vi "DAQmx Create Channel (TEDS-AI-Position-RVDT).vi"(0 "task in":refnum<k21>, 1 "maximum value":dbl=70.0 format="%0.2f", 2 "minimum value":dbl=-70.0 format="%0.2f", 3 "voltage excitation wire mode":i32(ring)=4 items=["4-Wire"=4, "5-Wire"=5, "6-Wire"=6], 5 "physical channels":tag, 6 "voltage excitation source":i32(ring)=10200 items=["Internal"=10200, "External"=10167, "None"=10230], 7 "name to assign":string, 8 "voltage excitation value":dbl=1.0, 9 "units":i32(ring)=10146 items=["Degrees"=10146, "Radians"=10273, "From Custom Scale"=10065], 10 "voltage excitation frequency":dbl=2500.0, 11 "error in":errorcluster, 12 "custom scale name":tag) -> (4 "task out":refnum<k21>, 15 "error out":errorcluster)   [LabVIEW 2018]
doc: "Creates channel(s) that use an RVDT to measure angular position. You must configure the physical channel(s) with TEDS information to use this VI."
uses:
  nilvaiu.dll
panel:
  # "input limits"
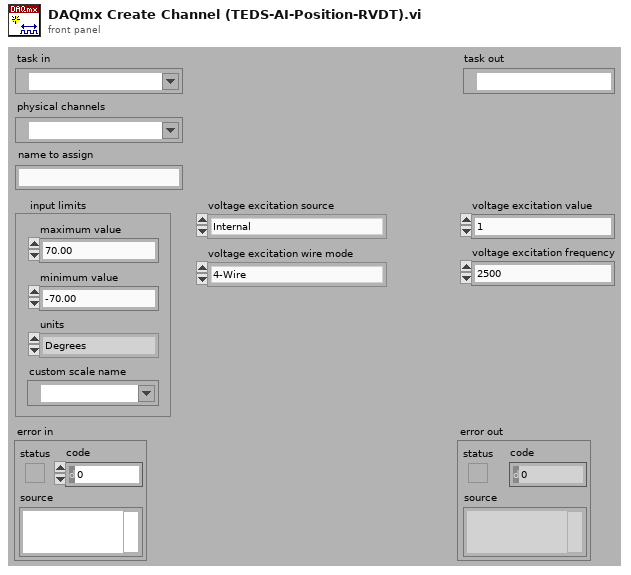
[diagram p1: front panel]
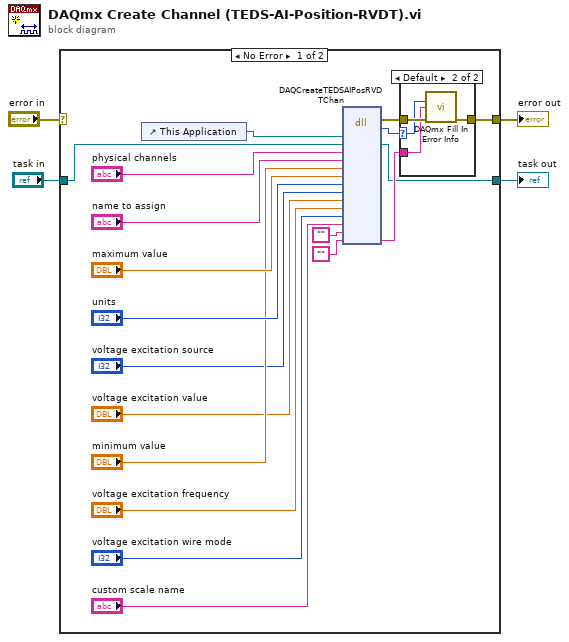
[diagram p0: block diagram]
diagram:
  n1 = case shown="No Error" "error in" {
    selector: "error in" -> [_ w30]
    tunnel: [w17 w30] -> w2
    tunnel: "task in" -> [w16 w29]
    tunnel: [w18 w29] -> w1
    frame No Error {
      n2 = control-ref of="This Application"() -> (w20:refnum<vi>)
      n3 = dll-call lib="nilvaiu.*" fn="DAQCreateTEDSAIPosRVDTChan"("lvAppRef"=w20, "refObjPtr"=w16, "physicalChannelName"="physical channels", "channelNameIn"="name to assign", "minVal"="minimum value", "maxVal"="maximum value", "units"="units", "voltageExcitSource"="voltage excitation source", "excitVal"="voltage excitation value", "excitFreq"="voltage excitation frequency", "ACExcitWireMode"="voltage excitation wire mode", "customScaleName"="custom scale name", "channelNamesOut"="", "extendedErrorInfo"="") -> (error out=w23:errorcluster, "return type"=w22:i32, "refObjPtr"=w18:refnum<k21>, "extendedErrorInfo"=w21:string)  [unwired: 15 in, 1 out]
      n4 = case shown="Default" w22 {
        selector: w22 -> [_ w26]
        tunnel: w23 -> [w24 w28]
        tunnel: [w24 w27] -> w17
        tunnel: w21 -> [_ w25]
        frame 0 {
        }
        frame Default {
          n5 = call "DAQmx Fill In Error Info.vi"("status code"=w26, "extended error info"=w25, "error in"=w28) -> ("error out"=w27:errorcluster)  [unwired: 1 in, 11 out]
        }
      }
    }
    frame Error {
    }
  }
  "error out" <- w2
  "task out" <- w1
